vi "GFITS_CheckID.vi"(6 "array name":string, 9 "expid":string, 10 "queue?":bool, 11 "value":string[][](array[string])) -> (2 "OK":bool, 3 "value out":string[][](array[string]))   [LabVIEW 2016]
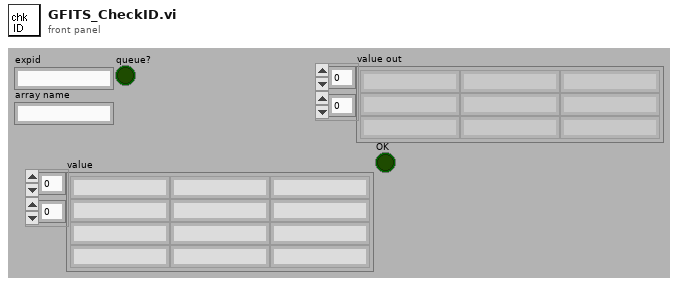
[diagram p1: front panel]
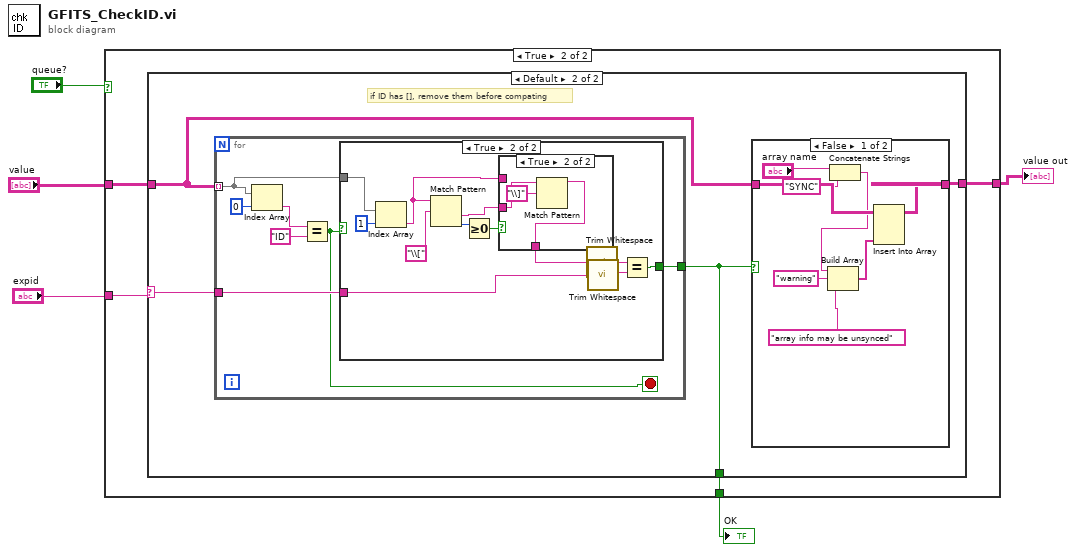
[diagram p0: block diagram]
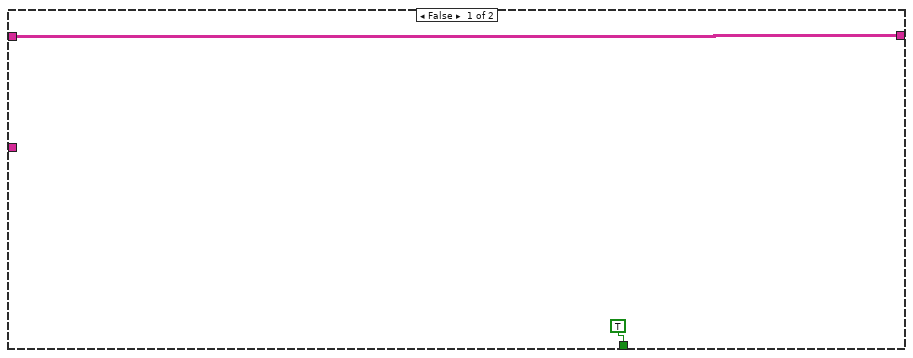
[diagram p2: hidden frame]
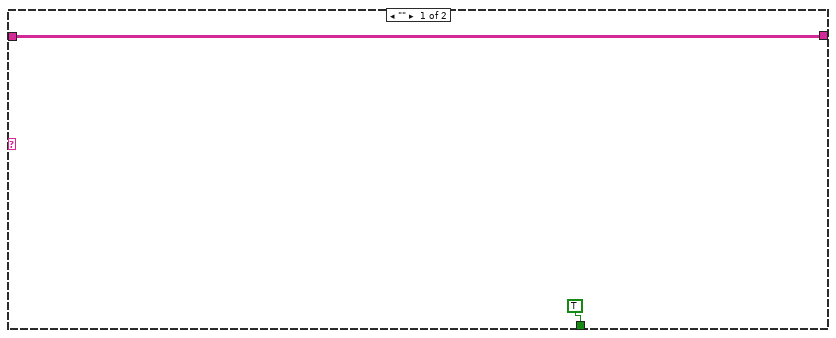
[diagram p3: hidden frame]
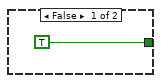
[diagram p5: hidden frame]
diagram:
  n1 = case shown="True" "queue?" {
    tunnel: "value" -> [w7 w11]
    tunnel: "expid" -> [_ w8]
    tunnel: [w7 w10] -> w1
    tunnel: [TRUE w9] -> w2
    frame False {
    }
    frame True {
      n2 = case shown="Default" w8 {
        selector: w8 -> [_ w14]
        tunnel: w11 -> [w13 w17]
        tunnel: [w13 w16] -> w10
        tunnel: [TRUE w15] -> w9
        frame "" {
        }
        frame Default {
          # "if ID has [], remove them before compating"
          n3 = for {
            tunnel: w17 -> [w29] mode=indexing
            tunnel: w14 -> [w30]
            tunnel: [w27] -> w15
            stop <- w28 stop-if-true
            n4 = Index Array(array=w29, index=0) -> (element=w32:string)
            n5 = Equal?(x=w32, y="ID") -> (x = y?=w28:bool)
            n6 = case shown="True" w28 {
              tunnel: w30 -> [_ w46]
              tunnel: w29 -> [_ w45]
              tunnel: [TRUE w43] -> w27
              frame False {
              }
              frame True {
                n7 = Index Array(array=w45, index=1) -> (element=w37:string)
                n8 = Match Pattern(string=w37, regular expression="\\[") -> (after substring=w35:string, offset past match=w39:i32)  [unwired: 3 out]
                n9 = Greater Or Equal To 0?(x=w39) -> (x >= 0?=w38:bool)
                n10 = case shown="True" w38 {
                  tunnel: w37 -> [w47 _]
                  tunnel: [w47 w48] -> w36
                  tunnel: w35 -> [_ w50]
                  frame False {
                  }
                  frame True {
                    n11 = Match Pattern(string=w50, regular expression="\\]") -> (before substring=w48:string)  [unwired: 4 out]
                  }
                }
                n12 = call <vilib>:"Trim Whitespace.vi"("string"=w36) -> ("trimmed string"=w41:string)  [unwired: 1 in]
                n13 = call <vilib>:"Trim Whitespace.vi"("string"=w46) -> ("trimmed string"=w42:string)  [unwired: 1 in]
                n14 = Equal?(x=w41, y=w42) -> (x = y?=w43:bool)
              }
            }
          }
          n15 = case shown="False" w15 {
            tunnel: w17 -> [w25 w26]
            tunnel: [w24 w26] -> w16
            frame False {
              n16 = Concatenate Strings("array name", "SYNC" ("string")) -> (w18:string)
              n17 = Build Array(w18, "warning" ("element"), "array info may be unsynced" ("element")) -> (w22:string[])
              n18 = Insert Into Array(array=w25, new element=w22) -> (w24:string[][])  [unwired: 2 in]
            }
            frame True {
            }
          }
        }
      }
    }
  }
  "value out" <- w1
  "OK" <- w2
